vi "vTab_9234_CHx1_9237_CHx3.vi"() -> ()   [LabVIEW 2018]
uses:
  <vilib>/Utility/sysdir.llb/System Directory Type.ctl
  <vilib>/express/express analysis/Spectral/Block/exnSpectralBlock spectral measurements peak poly.vi
  <vilib>/express/express analysis/Spectral/Block/exnSpectralBlock spectral measurements peak DDT.vi
  <vilib>/ErrorRing/Error Ring.xnode
  <vilib>/express/express analysis/Spectral/XNode/ExpressSpectralMeasurementsBlockNode.xnode
  <vilib>/Utility/config.llb/NI_LVConfig.lvlib
panel:
  out "RecFolder":string
  out "SVING 2":bool caption="存檔"
  out "SVING":bool caption="存檔"
  in  "Open Folder":bool
  in  "Enable Saving":bool
  out "Time":timestamp format="%<%Y/%m/%d   %H:%M:%S>T"
  in  "Tab Control":enum32{"觸發訊號", "參數設定"}(tab)
  out "Strain-CH4":dynamicdata(graph)
  out "Strain-CH3":dynamicdata(graph)
  out "Strain-CH2":dynamicdata(graph)
  out "Strain-CH1":dynamicdata(graph)
  out "Acc_Sig":dynamicdata(graph)
  in  "ACCFFT":bool
  in  "DAQ2 (請選取 NI 9237 )":tag="cDAQ1Mod1"
  out "DAQ Stoped 2":bool caption="DAQ Stoped"
  in  "Sample Rate":dbl=10000.0 format="%#_13g"
  in  "Samples to Read":i32=10000
  in  "Lower Cut-Off (Hz)":dbl=100.0
  in  "DAQ1 (請選取 NI 9234 )":tag="cDAQ1Mod1"
  in  "ABORT":bool
  in  "Run":bool
  out "DAQ Stoped":bool
  in  "PAUSE":bool
  out "DAQ Error":errorcluster
  out "DAQ1":i32
  out "DAQ1":i32(slide) scale=0.0..100.0
  in  "Sample Rate":dbl=10000.0 format="%#_13g"
  in  "Samples to Read":i32=10000
  out "DAQ2_Preview":dynamicdata(graph)
  out "DAQ1_Preview":dynamicdata(graph)
  out "DAQ2":i32(slide) scale=0.0..100.0
  out "DAQ2":i32
  # "使用前請至 參數設置 設定"
  # "本頁畫面顯示為 觸發後訊號"
  # "FFT Filter by useing High-pass with Lower Cut-Off (Hz)"
  # "擷取卡設定"
  # "擷取卡設定"
  # "(系統開啟後修改無效)"
  # "(系統開啟後修改無效)"
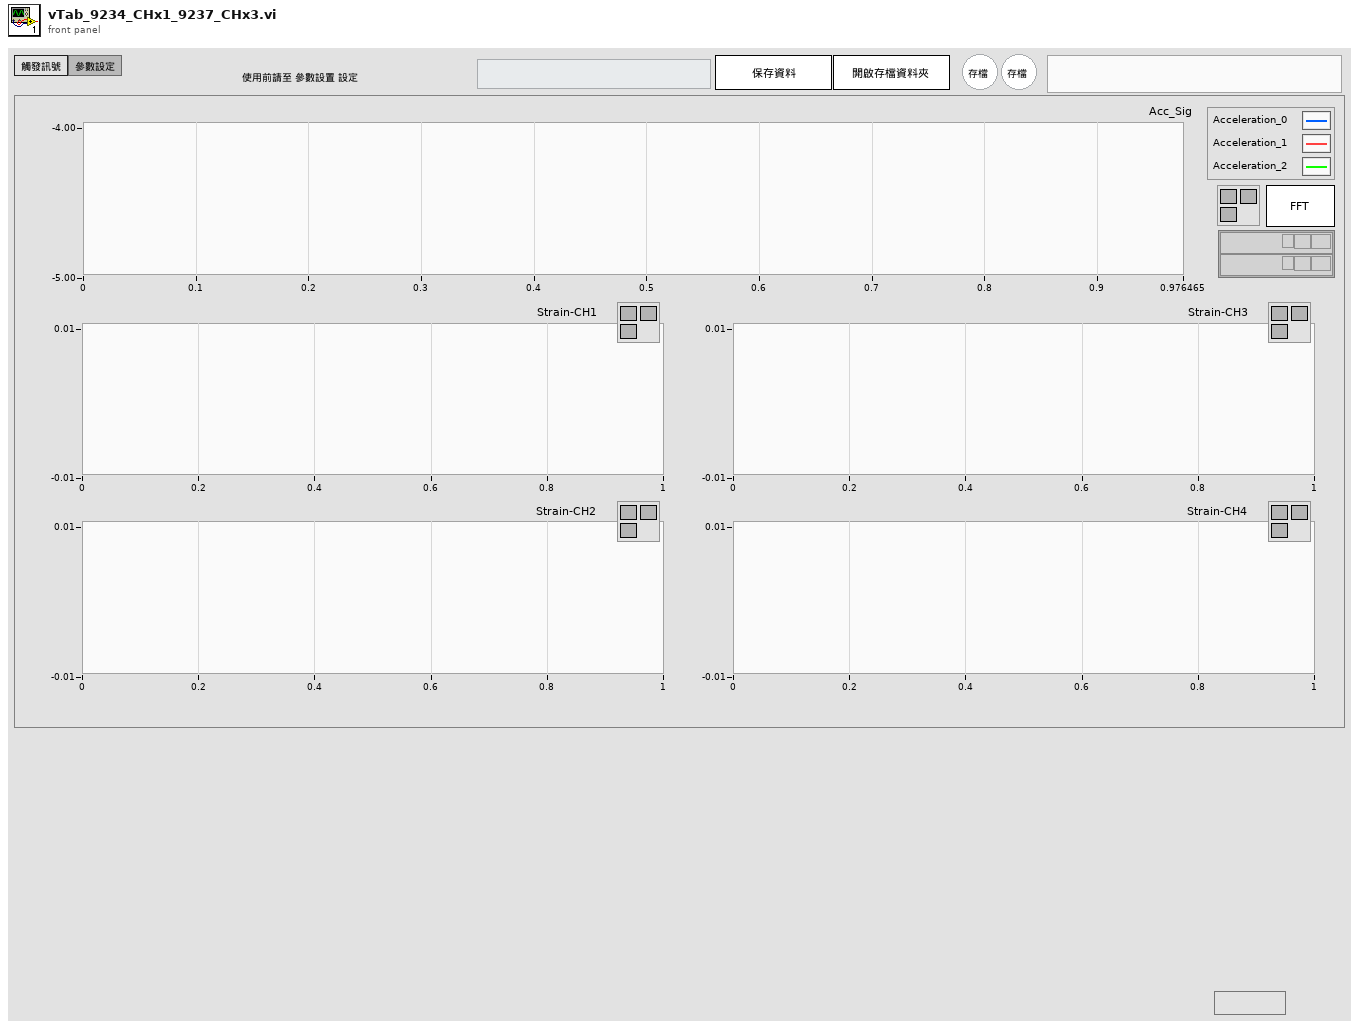
[diagram p1: front panel]
types:
  T1 = typedef "NI_LVConfig.lvlib/Config Data RefNum.ctl" = refnum<k1>
  T2 = enum8{"Enabled", "Disabled", "Disabled and Grayed Out"}
  T3 = cluster{"averaging mode":u16, "weighting mode":u16, "number of averages":u32}
  T4 = cluster{"dB On (F)":bool, "unwrap phase (F)":bool, "convert to degree (F)":bool}
  T5 = typedef "System Directory Type.ctl" = i32
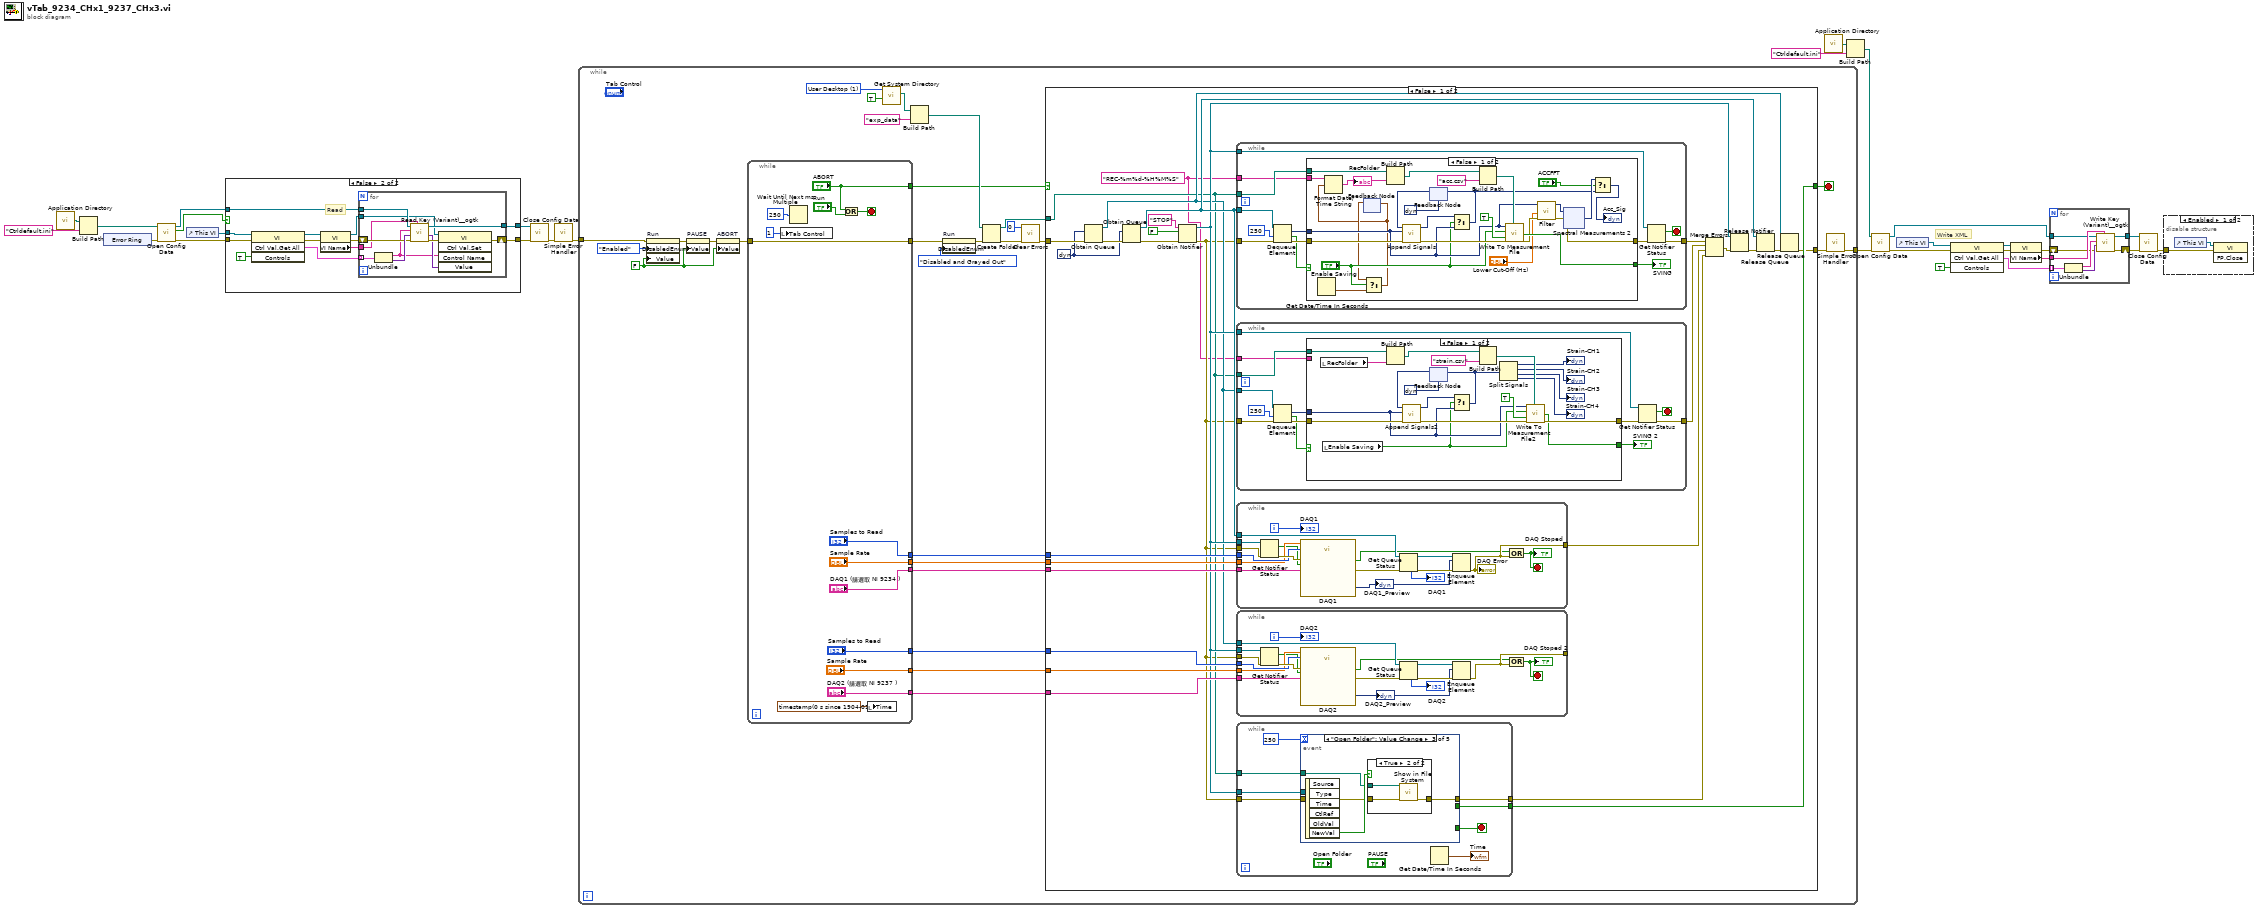
[diagram p0: block diagram]
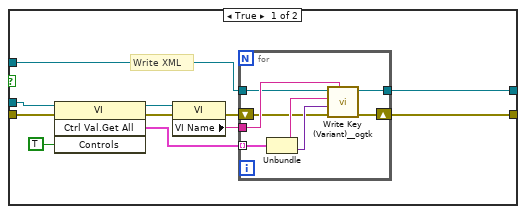
[diagram p2: hidden frame]
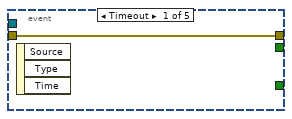
[diagram p6: hidden frame]
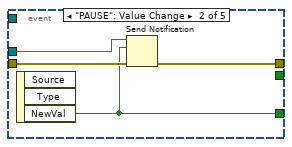
[diagram p7: hidden frame]
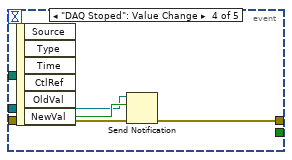
[diagram p9: hidden frame]
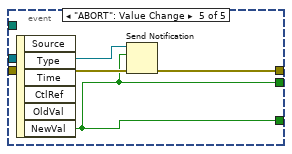
[diagram p10: hidden frame]
diagram:
  # "Write XML"
  n1 = call <vilib>:"Application Directory.vi"() -> ("Application Directory"=w1:path)
  n2 = Build Path(base path=w1, name or relative path="Ctrldefault.ini") -> (appended path=w28:path)
  n3 = xnode "Error Ring"() -> ("error out"=w20:errorcluster)
  n4 = call <vilib>:"Open Config Data.vi"("error in (no error)"=w20, "configuration file path"=w28) -> ("error out"=w25:errorcluster, "file created?"=w21:bool, "refnum"=w18:T1)  [unwired: 7 in]
  n5 = control-ref of="This VI"() -> (w19:refnum<vi>)
  n6 = case shown="False" w21 {
    tunnel: [w33 w53] -> w26
    tunnel: w25 -> [w31 w51]
    tunnel: [w29 w49] -> w24
    tunnel: w19 -> [w32 w52]
    tunnel: w18 -> [w34 w54]
    frame True {
      # "Write XML"
      n7 = invoke class="VI" method="Ctrl Val.Get All"(reference=w32, error in=w31, "Controls"=TRUE) -> (reference out=w38:refnum<vi>, error out=w37:errorcluster, "Get All Control Values Variant"=w39:cluster{"Name":string, "Variant Data":variant}[])  [unwired: 1 in, 1 out]
      n8 = property class="VI"(reference=w38, error in=w37) -> (error out=w30:errorcluster, "VI Name"=w36:string)  [unwired: 1 out]
      n9 = for {
        tunnel: w39 -> [w47] mode=indexing
        tunnel: w36 -> [w46]
        tunnel: w34 -> [w44]
        shift-right: [w43] -> w33
        shift-left: w30 -> [w41]
        tunnel: [w40] -> w29
        n10 = Unbundle(w47) -> ("Name"=w45:string, "Variant Data"=w42:variant)
        n11 = call <userlib>:"Write Key (Variant)__ogtk.vi"("section"=w46, "error in (no error)"=w41, "key-value"=w42, "key (optional)"=w45, "refnum"=w44) -> ("error out"=w43:errorcluster, "refnum out"=w40:T1)  [unwired: 5 in]
      }
    }
    frame False {
      # "Read"
      n12 = invoke class="VI" method="Ctrl Val.Get All"(reference=w52, error in=w51, "Controls"=TRUE) -> (reference out=w58:refnum<vi>, error out=w57:errorcluster, "Get All Control Values Variant"=w59:cluster{"Name":string, "Variant Data":variant}[])  [unwired: 1 in, 1 out]
      n13 = property class="VI"(reference=w58, error in=w57) -> (reference out=w48:refnum<vi>, error out=w50:errorcluster, "VI Name"=w56:string)
      n14 = for {
        tunnel: w59 -> [w70] mode=indexing
        tunnel: w56 -> [w63]
        tunnel: w54 -> [w69]
        shift-right: [w64] -> w53
        shift-left: w50 -> [w67]
        tunnel: [w66] -> w49
        tunnel: w48 -> [w62]
        n15 = Unbundle(w70) -> ("Name"=w60:string, "Variant Data"=w68:variant)
        n16 = call <userlib>:"Read Key (Variant)__ogtk.vi"("section"=w63, "error in (no error)"=w67, "type"=w68, "key (optional)"=w60, "refnum"=w69) -> ("error out"=w65:errorcluster, "key-value"=w61:variant, "refnum out"=w66:T1)  [unwired: 3 in, 1 out]
        n17 = invoke class="VI" method="Ctrl Val.Set"(reference=w62, error in=w65, "Control Name"=w60, "Value"=w61) -> (error out=w64:errorcluster)  [unwired: 1 in, 4 out]
      }
    }
  }
  n18 = call <vilib>:"Close Config Data.vi"("error in (no error)"=w26, "refnum"=w24) -> ("error out"=w23:errorcluster)  [unwired: 8 in, 1 out]
  n19 = call <vilib>:"Simple Error Handler.vi"("error in (no error)"=w23) -> ("error out"=w22:errorcluster)  [unwired: 4 in, 4 out]
  n20 = while {
    tunnel: [w98] -> w4
    tunnel: w22 -> [w76]
    stop <- w79 stop-if-true
    w87 = T5 1 items=["User Home"=0, "User Desktop"=1, "User Documents"=2, "User Application Data"=3, "User Preferences"=4, "User Temporary"=5, "Public Documents"=6, "Public Application Data"=7, "Public Preferences"=8, "Public Cache"=13, "System Core Libraries"=9, "System Installed Libraries"=10, "Application Files"=11, "Boot Volume Root"=12] ("system directory type")
    w92 = FALSE ("stop 3")
    n21 = property on="Run" class="Bool (strict)"(error in=w76, "DisabledEnum"=T2."Enabled" ("Disabled"), "Value"=w92) -> (error out=w95:errorcluster)  [unwired: 1 in, 1 out]
    n22 = property on="PAUSE" class="Bool (strict)"(error in=w95, "Value"=w92) -> (error out=w94:errorcluster)  [unwired: 1 in, 1 out]
    n23 = property on="ABORT" class="Bool (strict)"(error in=w94, "Value"=w92) -> (error out=w93:errorcluster)  [unwired: 1 in, 1 out]
    n24 = while {
      tunnel: [w287] -> w75
      tunnel: w93 -> [w287]
      tunnel: ["Samples to Read"] -> w78
      tunnel: ["Sample Rate"] -> w82
      tunnel: ["DAQ1 (請選取 NI 9234 )"] -> w80
      tunnel: ["ABORT"] -> w74
      tunnel: ["DAQ2 (請選取 NI 9237 )"] -> w73
      tunnel: ["Sample Rate"] -> w72
      tunnel: ["Samples to Read"] -> w71
      stop <- w280 stop-if-true
      n25 = local write "Tab Control"(1) -> ()
      n26 = Wait Until Next ms Multiple(millisecond multiple=u32 250) -> ()  [unwired: 1 out]
      n27 = Or(x="ABORT", y="Run") -> (x .or. y?=w280:bool)
      n28 = local write "Time"(timestamp(0 s since 1904-01-01) ("Time 2")) -> ()
    }
    n29 = call <vilib>:"Get System Directory.vi"("create directory if not found? (F)"=TRUE, "system directory type"=w87) -> ("system directory"=w89:path)  [unwired: 9 in]
    n30 = Build Path(base path=w89, name or relative path="exp_data") -> (appended path=w86:path)
    n31 = property on="Run" class="Bool (strict)"(error in=w75, "DisabledEnum"=T2."Disabled and Grayed Out" ("Disabled")) -> (error out=w90:errorcluster)  [unwired: 1 in, 1 out]
    n32 = Create Folder(path (use dialog)=w86, error in=w90) -> (created path=w77:path, error out=w84:errorcluster)  [unwired: 1 in, 1 out]
    n33 = call <vilib>:"Clear Errors.vi"("error in (no error)"=w84, "specific error code to clear (0: all)"=0) -> ("error out"=w83:errorcluster)  [unwired: 4 in, 1 out]
    n34 = case shown="False" w74 {
      selector: w74 -> [_ w273]
      tunnel: w83 -> [w119 w274]
      tunnel: w82 -> [w118 _]
      tunnel: [w106 w274] -> w81
      tunnel: w80 -> [w115 _]
      tunnel: [w114 w273] -> w79
      tunnel: w78 -> [w113 _]
      tunnel: w77 -> [w101 _]
      tunnel: w73 -> [w111 _]
      tunnel: w72 -> [w110 _]
      tunnel: w71 -> [w109 _]
      frame False {
        w99 = "REC-%m%d-%H%M%S" ("time format string (%c)")
        w108 = dynamicdata [] ("DAQ1_Preview 2")
        n35 = Obtain Queue(element data type=w108) -> (queue out=w102:refnum<queue>)  [unwired: 4 in, 2 out]
        n36 = Obtain Queue(element data type=w108, error in (no error)=w119) -> (queue out=w112:refnum<queue>, error out=w122:errorcluster)  [unwired: 3 in, 1 out]
        n37 = Obtain Notifier(name (unnamed)="STOP", notification data type=FALSE, error in (no error)=w122) -> (notifier out=w103:refnum<notifier>, error out=w100:errorcluster)  [unwired: 1 in, 1 out]
        n38 = while {
          tunnel: w112 -> [w180]
          tunnel: w100 -> [w187]
          tunnel: [w183] -> w105
          tunnel: w103 -> [w181]
          tunnel: w101 -> [w178]
          tunnel: w99 -> [w176]
          stop <- w182 stop-if-true
          n39 = Dequeue Element(queue=w180, timeout in ms (-1)=250, error in (no error)=w187) -> (element=w186:dynamicdata, timed out?=w179:bool, error out=w185:errorcluster)  [unwired: 1 out]
          n40 = case shown="False" w179 {
            tunnel: w186 -> [w203 _]
            tunnel: w185 -> [w211 w226]
            tunnel: [w204 w226] -> w184
            tunnel: w178 -> [w193 _]
            tunnel: [w207 _] -> w177
            tunnel: w176 -> [w195 _]
            frame False {
              n41 = Get Date/Time In Seconds() -> (seconds since 1Jan1904=w191:timestamp)
              n42 = feedback #1() -> (w190:timestamp)  [unwired: 1 in]
              n43 = Select(t=w190, s="Enable Saving", f=w191) -> (s? t:f=w189:timestamp)
              n44 = Format Date/Time String(time format string (%c)=w195, seconds (now)=w189) -> (date/time string=w194:string)  [unwired: 1 in]
              "RecFolder" <- w194
              n45 = feedback-in #1(w189) -> ()
              n46 = Build Path(base path=w193, name or relative path=w194) -> (appended path=w196:path)
              n47 = feedback #2(dynamicdata [] ("Waveform Graph")) -> (w214:dynamicdata)
              n48 = call "Append Signals"("error in (no error)"=w211, "Input Signal B"=w203, "Input Signal A"=w214) -> ("error out"=w210:errorcluster, "Appended Signals"=w213:dynamicdata)  [unwired: 7 in]
              n49 = Select(t=w213, s="Enable Saving", f=w203) -> (s? t:f=w198:dynamicdata)
              n50 = feedback-in #2(w198) -> ()
              n51 = Build Path(base path=w196, name or relative path="acc.csv") -> (appended path=w208:path)
              n52 = call "Write To Measurement File"("Signals"=w203, "Enable"="Enable Saving", "new_file"=TRUE, "error in (no error)"=w210, "Filename"=w208) -> ("Saving Data"=w207:bool, "error out"=w205:errorcluster)  [unwired: 12 in, 1 out]
              n53 = call "Filter"("error in (no error)"=w205, "Lower Cut-Off"="Lower Cut-Off (Hz)", "Signal"=w203) -> ("error out"=w206:errorcluster, "Filtered Signal"=w202:dynamicdata)  [unwired: 7 in]
              n54 = xnode ("Spectral Measurements 2")("Signals"=w202, "error in (no error)"=w206) -> ("FFT - (Peak)"=w200:dynamicdata, "error out"=w204:errorcluster)  [unwired: 1 out]
              n55 = Select(t=w200, s="ACCFFT", f=w198) -> (s? t:f=→"Acc_Sig":dynamicdata)
            }
            frame True {
            }
          }
          "SVING" <- w177
          n56 = Get Notifier Status(notifier=w181, error in (no error)=w184) -> (current notification=w182:bool, error out=w183:errorcluster)  [unwired: 3 out]
        }
        n57 = while {
          tunnel: w102 -> [w129]
          tunnel: w100 -> [w136]
          tunnel: [w132] -> w104
          tunnel: w103 -> [w130]
          tunnel: w101 -> [w127]
          tunnel: w99 -> [w125]
          stop <- w131 stop-if-true
          n58 = Dequeue Element(queue=w129, timeout in ms (-1)=250, error in (no error)=w136) -> (element=w135:dynamicdata, timed out?=w128:bool, error out=w134:errorcluster)  [unwired: 1 out]
          n59 = case shown="False" w128 {
            tunnel: w135 -> [w151 _]
            tunnel: w134 -> [w153 w158]
            tunnel: [w148 w158] -> w133
            tunnel: w127 -> [w140 _]
            tunnel: [w142 _] -> w126
            tunnel: w125 -> [_ _]
            frame False {
              n60 = local read "RecFolder"() -> (w138:string)
              n61 = local read "Enable Saving"() -> (w139:bool)
              n62 = Build Path(base path=w140, name or relative path=w138) -> (appended path=w141:path)
              n63 = feedback #3(dynamicdata [] ("Waveform Graph")) -> (w156:dynamicdata)
              n64 = call "Append Signals2"("error in (no error)"=w153, "Input Signal B"=w151, "Input Signal A"=w156) -> ("error out"=w152:errorcluster, "Appended Signals"=w155:dynamicdata)  [unwired: 7 in]
              n65 = Select(t=w155, s=w139, f=w151) -> (s? t:f=w147:dynamicdata)
              n66 = feedback-in #3(w147) -> ()
              n67 = Build Path(base path=w141, name or relative path="strain.csv") -> (appended path=w149:path)
              n68 = Split Signals(w147) -> (→"Strain-CH1":dynamicdata, →"Strain-CH2":dynamicdata, →"Strain-CH3":dynamicdata, →"Strain-CH4":dynamicdata)  [unwired: 4 in]
              n69 = call "Write To Measurement File2"("Signals"=w151, "Enable"=w139, "new_file"=TRUE, "error in (no error)"=w152, "Filename"=w149) -> ("Saving Data"=w142:bool, "error out"=w148:errorcluster)  [unwired: 12 in, 1 out]
            }
            frame True {
            }
          }
          "SVING 2" <- w126
          n70 = Get Notifier Status(notifier=w130, error in (no error)=w133) -> (current notification=w131:bool, error out=w132:errorcluster)  [unwired: 3 out]
        }
        n71 = while {
          tunnel: w112 -> [w241]
          tunnel: [w233] -> w123
          tunnel: w100 -> [w237]
          tunnel: w103 -> [w235]
          tunnel: w113 -> [w232]
          tunnel: w118 -> [w231]
          tunnel: w115 -> [w227]
          i -> [w243]
          stop <- w234 stop-if-true
          n72 = Get Notifier Status(notifier=w235, error in (no error)=w237) -> (current notification=w230:bool, error out=w236:errorcluster)  [unwired: 3 out]
          n73 = call "DAQ1"("rate"=w231, "number of samples"=w232, "error in"=w236, "stop (F)"=w230, "device name"=w227) -> ("data"=w228:dynamicdata, "stopped"=w229:bool, "error out"=w238:errorcluster)  [unwired: 11 in, 1 out]
          "DAQ1_Preview" <- w228
          n74 = Get Queue Status(queue=w241, error in (no error)=w238) -> (queue out=w240:refnum<queue>, error out=w239:errorcluster, # elements in queue=→"DAQ1":i32)  [unwired: 1 in, 5 out]
          n75 = Enqueue Element(queue=w240, element=w228, error in (no error)=w239) -> (error out=w233:errorcluster)  [unwired: 1 in, 2 out]
          "DAQ Error" <- w233
          n76 = Compound Arithmetic op=OR(w229, w233) -> (w234:bool)
          "DAQ Stoped" <- w234
          "DAQ1" <- w243
        }
        n77 = while {
          tunnel: w102 -> [w173]
          tunnel: [w166] -> _
          tunnel: w100 -> [w169]
          tunnel: w103 -> [w167]
          tunnel: w109 -> [w165]
          tunnel: w110 -> [w164]
          tunnel: w111 -> [w160]
          i -> [w175]
          stop <- w159 stop-if-true
          n78 = Get Notifier Status(notifier=w167, error in (no error)=w169) -> (current notification=w163:bool, error out=w168:errorcluster)  [unwired: 3 out]
          n79 = call "DAQ2"("rate"=w164, "number of samples"=w165, "error in"=w168, "stop (F)"=w163, "device name"=w160) -> ("data"=w161:dynamicdata, "stopped"=w162:bool, "error out"=w170:errorcluster)  [unwired: 11 in, 1 out]
          "DAQ2_Preview" <- w161
          n80 = Get Queue Status(queue=w173, error in (no error)=w170) -> (queue out=w172:refnum<queue>, error out=w171:errorcluster, # elements in queue=→"DAQ2":i32)  [unwired: 1 in, 5 out]
          n81 = Enqueue Element(queue=w172, element=w161, error in (no error)=w171) -> (error out=w166:errorcluster)  [unwired: 1 in, 2 out]
          n82 = Compound Arithmetic op=OR(w162, w166) -> (w159:bool)
          "DAQ Stoped 2" <- w159
          "DAQ2" <- w175
        }
        n83 = while {
          tunnel: w100 -> [w251]
          tunnel: [w250] -> w124
          tunnel: w103 -> [w248]
          tunnel: [w245] -> w114
          tunnel: w101 -> [w244]
          stop <- w246 stop-if-true
          n84 = event shown="[2] \"Open Folder\": Value Change" {
            selector: _ -> [_ _ _ _ _]
            dyn-events: _ -> [_ _ _ _ _]
            timeout: 250 -> [_ _ _ _ _]
            tunnel: w251 -> [w252 w256 w259 w268 w272]
            tunnel: [w252 w255 w257 w265 w271] -> w250
            tunnel: w248 -> [_ w254 _ w266 w270]
            tunnel: [_ w253 _ _ w269] -> w246
            tunnel: [_ _ _ _ w269] -> w245
            tunnel: w244 -> [_ _ w258 _ _]
            event Timeout {
              n85 = event-data() -> ()  [unwired: 1 in, 3 out]
            }
            event "PAUSE": Value Change {
              n86 = event-data() -> ("NewVal"=w253:bool)  [unwired: 1 in, 2 out]
              n87 = Send Notification(notification=w253, notifier=w254, error in (no error)=w256) -> (error out=w255:errorcluster)  [unwired: 1 out]
            }
            event "Open Folder": Value Change {
              n88 = event-data() -> ("NewVal"=w260:bool)  [unwired: 1 in, 5 out]
              n89 = case shown="True" w260 {
                tunnel: w259 -> [w261 w264]
                tunnel: w258 -> [_ w263]
                tunnel: [w261 w262] -> w257
                frame False {
                }
                frame True {
                  n90 = call <vilib>:"Show in File System.vi"("error in (no error)"=w264, "file or directory path"=w263) -> ("error out"=w262:errorcluster)  [unwired: 9 in]
                }
              }
            }
            event "DAQ Stoped": Value Change {
              n91 = event-data() -> ("NewVal"=w267:bool)  [unwired: 1 in, 5 out]
              n92 = Send Notification(notification=w267, notifier=w266, error in (no error)=w268) -> (error out=w265:errorcluster)  [unwired: 1 out]
            }
            event "ABORT": Value Change {
              n93 = event-data() -> ("NewVal"=w269:bool)  [unwired: 1 in, 5 out]
              n94 = Send Notification(notification=w269, notifier=w270, error in (no error)=w272) -> (error out=w271:errorcluster)  [unwired: 1 out]
            }
          }
          n95 = Get Date/Time In Seconds() -> (seconds since 1Jan1904=→"Time":timestamp)
        }
        n96 = Merge Errors(w105, w104, w123, w124) -> (w116:errorcluster)
        n97 = Release Notifier(notifier=w103, error in (no error)=w116) -> (error out=w117:errorcluster)  [unwired: 1 in, 2 out]
        n98 = Release Queue(queue=w112, error in (no error)=w117) -> (error out=w107:errorcluster)  [unwired: 1 in, 2 out]
        n99 = Release Queue(queue=w102, error in (no error)=w107) -> (error out=w106:errorcluster)  [unwired: 1 in, 2 out]
      }
      frame True {
      }
    }
    n100 = call <vilib>:"Simple Error Handler.vi"("error in (no error)"=w81) -> ("error out"=w98:errorcluster)  [unwired: 4 in, 4 out]
  }
  n101 = call <vilib>:"Application Directory.vi"() -> ("Application Directory"=w2:path)
  n102 = Build Path(base path=w2, name or relative path="Ctrldefault.ini") -> (appended path=w11:path)
  n103 = call <vilib>:"Open Config Data.vi"("error in (no error)"=w4, "configuration file path"=w11) -> ("error out"=w14:errorcluster, "refnum"=w17:T1)  [unwired: 7 in, 1 out]
  n104 = control-ref of="This VI"() -> (w16:refnum<vi>)
  n105 = invoke class="VI" method="Ctrl Val.Get All"(reference=w16, error in=w14, "Controls"=TRUE) -> (reference out=w9:refnum<vi>, error out=w8:errorcluster, "Get All Control Values Variant"=w10:cluster{"Name":string, "Variant Data":variant}[])  [unwired: 1 in, 1 out]
  n106 = property class="VI"(reference=w9, error in=w8) -> (error out=w5:errorcluster, "VI Name"=w7:string)  [unwired: 1 out]
  n107 = for {
    tunnel: w10 -> [w295] mode=indexing
    tunnel: w7 -> [w294]
    tunnel: w17 -> [w292]
    shift-right: [w291] -> w13
    shift-left: w5 -> [w289]
    tunnel: [w288] -> w15
    n108 = Unbundle(w295) -> ("Name"=w293:string, "Variant Data"=w290:variant)
    n109 = call <userlib>:"Write Key (Variant)__ogtk.vi"("section"=w294, "error in (no error)"=w289, "key-value"=w290, "key (optional)"=w293, "refnum"=w292) -> ("error out"=w291:errorcluster, "refnum out"=w288:T1)  [unwired: 5 in]
  }
  n110 = call <vilib>:"Close Config Data.vi"("error in (no error)"=w13, "refnum"=w15) -> ("error out"=w3:errorcluster)  [unwired: 8 in, 1 out]
  n111 = disable-structure shown="Enabled" {
    disable-tunnel: w3 -> [w296 _]
    frame Enabled {
      n112 = control-ref of="This VI"() -> (w297:refnum<vi>)
      n113 = invoke class="VI" method="FP.Close"(reference=w297, error in=w296) -> ()  [unwired: 1 in, 3 out]
    }
    frame Disabled {
    }
  }
